vi "Bessel IIR Filter Design.vi"() -> ()   [LabVIEW 2023]
doc: "Demonstrates how to use the DFD Bessel Design VI to design a digital Bessel filter with the filter specifications you entered. A Bessel filter has an approximately linear phase in the passband.\n\nComplete the following steps to use this VI.\n1) Run the VI.\n2) Change the specifications and observe the changes in the frequency response.\n3) Click the <B>STOP</B> button to stop this VI."
uses:
  <vilib>/addons/Digital Filter Design/_Objects.llb/DFD Phase Setting.ctl
  <vilib>/addons/Digital Filter Design/Analysis.llb/DFD Plot Freq Response (Linear-Spaced).vi
  <vilib>/addons/Digital Filter Design/NI_DigFilterLicensed.lvlib
panel:
  in  "stop":bool
  out "Error Message":string
  out "Frequency Response":cluster{"f0":dbl, "df":dbl, "values":dbl[]}[](graph)
  in  "Filter Type":T1(ring)
  in  "Sampling Frequency [Hz]":dbl=1.0 format="%.2f"
  in  "Low Cutoff Frequency [Hz]":dbl=0.12
  in  "High Cutoff Frequency [Hz]":dbl=0.45
  in  "Order":i32=2
  # "Select Help>>Show Context Help and move the cursor over the VI icon for more information."
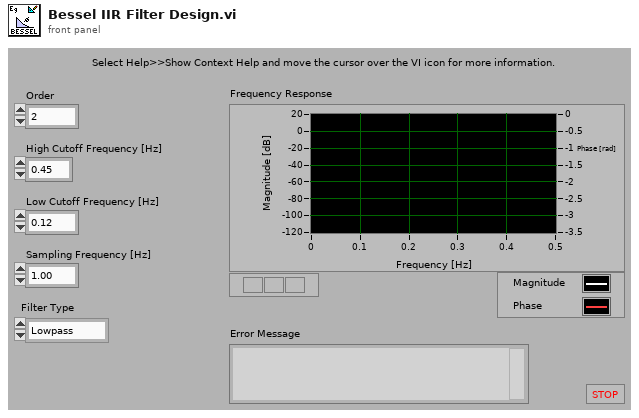
[diagram p1: front panel]
types:
  T1 = enum16{"Lowpass", "Highpass", "Bandpass", "Bandstop"}
  T2 = typedef "NI_DigFilterLicensed.lvlib/DFD Phase Setting.ctl" = cluster{"unwrap? (F)":bool, "degree? (F)":bool}
  T3 = typedef "NI_DigFilterLicensed.lvlib/DFD Filter Obj.ctl" = cluster{"mSRate_Fs":dbl, "mSRate_Version":string, "mSRate_Comments":string, "mSRate_OrgCoef":T4, "mSRate_CurCoef":T4, "mSRate_Quantized?":bool, "mSRate_QCoef":T4, "mSRate_QSettings":T6[], "mSRate_Order":i32, "mSRate_Scaling":cluster{"mSRate_ScaleByPowerOf2?":bool, "mSRate_ScaleType":T8}}
  T4 = typedef "NI_DigFilterLicensed.lvlib/DFD Filter Coef.ctl" = cluster{"type":T5, "gain":dbl, "coef a (k)":dbl[], "coef b (v)":dbl[]}
  T5 = typedef "NI_DigFilterLicensed.lvlib/DFD Filter Structure Type Selector.ctl" = enum16{"Undefined", "FIR Direct Form", "FIR Direct Form Transposed", "FIR Symmetric", "FIR Antisymmetric", "IIR Direct Form I", "IIR Direct Form I Transposed", "IIR Direct Form II", "IIR Direct Form II Transposed", "IIR Cascaded Second Order Sections Form I", "IIR Cascaded Second Order Sections Form I Transposed", "IIR Cascaded Second Order Sections Form II", "IIR Cascaded Second Order Sections Form II Transposed", "Lattice Allpass (basic sections)", "Lattice Allpass (one multiplier sections)", "Lattice Allpass (normalized sections)", "Lattice AR (basic sections)", "Lattice AR (one multiplier sections)", "Lattice AR (normalized sections)", "Lattice MA (minimum phase)", "Lattice MA (maximum phase)", "Lattice ARMA (basic sections)", "Lattice ARMA (one multiplier sections)", "Lattice ARMA (normalized sections)"}
  T6 = typedef "NI_DigFilterLicensed.lvlib/dfd_Internal Quantization Settings.ctl" = cluster{"source":T7, "wl":i16, "iwl":i16, "overflow mode":enum16{"Saturation", "Wrap"}, "rounding mode":enum16{"Nearest", "Truncation"}, "signed?":bool}
  T7 = typedef "NI_DigFilterLicensed.lvlib/dfd_Internal Quantization Srcs.ctl" = u16
  T8 = typedef "NI_DigFilterLicensed.lvlib/DFD Coef Norm Type.ctl" = enum16{"No Norm", "Time Domain 1-Norm", "Time Domain 2-Norm", "Time Domain Inf-Norm"}
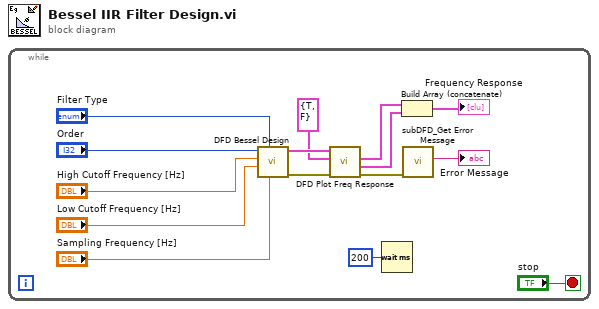
[diagram p0: block diagram]
diagram:
  n1 = while {
    stop <- "stop" stop-if-true
    n2 = call <vilib>:"DFD Bessel Design.vi"("fs [Hz]"="Sampling Frequency [Hz]", "filter type"="Filter Type", "low cutoff freq [Hz]"="Low Cutoff Frequency [Hz]", "high cutoff freq [Hz]"="High Cutoff Frequency [Hz]", "order"="Order") -> ("error out"=w11:errorcluster, "filter out"=w12:T3)  [unwired: 1 in, 4 out]
    n3 = call-poly <vilib>:"DFD Plot Freq Response.vi"("error in (no error)"=w11, "phase view"=T2 {"unwrap? (F)"=TRUE, "degree? (F)"=FALSE}, "filter in"=w12) -> ("error out"=w8:errorcluster, "phase response"=w3:cluster{"f0":dbl, "df":dbl, "values":dbl[]}[], "magnitude response"=w4:cluster{"f0":dbl, "df":dbl, "values":dbl[]}[])  [unwired: 5 in, 1 out]
    n4 = Wait (ms)(milliseconds to wait=u32 200) -> ()  [unwired: 1 out]
    n5 = Build Array (concatenate)(w4, w3) -> (→"Frequency Response":cluster{"f0":dbl, "df":dbl, "values":dbl[]}[])
    n6 = call <vilib>:"subDFD_Get Error Message.vi"("error in (no error)"=w8) -> ("Error Message"=→"Error Message":string)  [unwired: 10 out]
  }
